vi "Run.vi"(8 "error in (no error)":errorcluster, 11 "Event in":refnum<class "Event.lvclass">) -> (0 "error out":errorcluster, 3 "Event out":refnum<class "Event.lvclass">)   [LabVIEW 2012, in "MDSplus.lvlib" / "Event.lvclass"]
doc: "Method run is called upon reception of the event with the associated name, specified in the constructor. The default implementation is void, and it will be likely overridden by subclasses."
uses:
  <vilib>/MDSplus/Classes/Event_Class/Event.lvclass
  <vilib>/MDSplus/MDSobjectsLVShr_64.dll
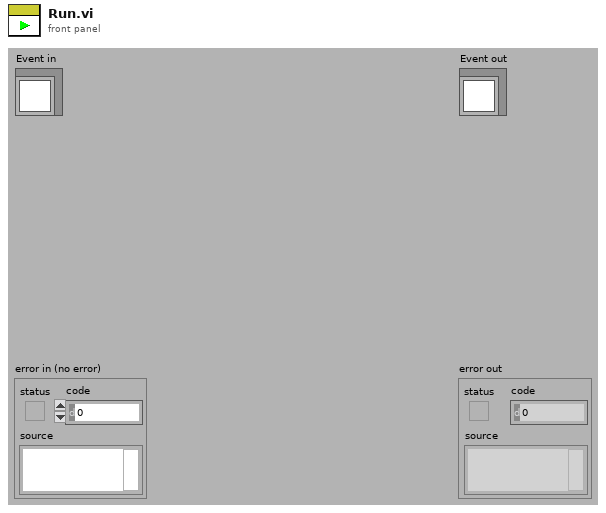
[diagram p1: front panel]
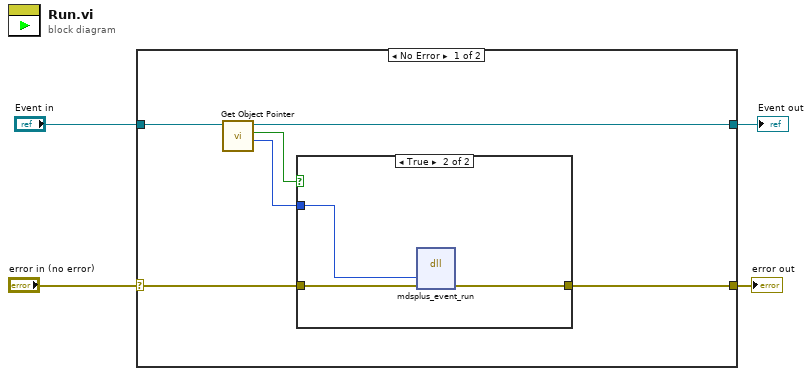
[diagram p0: block diagram]
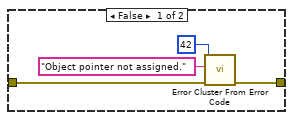
[diagram p2: hidden frame]
diagram:
  n1 = case shown="No Error" "error in (no error)" {
    selector: "error in (no error)" -> [w7 w19]
    tunnel: [w8 w19] -> w3
    tunnel: [w9 w18] -> w1
    tunnel: "Event in" -> [w10 w18]
    frame No Error {
      n2 = call-dynamic "Get Object Pointer.vi"("Event in"=w10) -> ("Object Pointer"=w5:i64, "Assigned object pointer?"=w6:bool, "Event out"=w9:refnum<class "Event.lvclass">)  [unwired: 8 in]
      n3 = case shown="True" w6 {
        tunnel: [w11 w17] -> w8
        tunnel: w7 -> [w12 w16]
        tunnel: w5 -> [_ w15]
        frame False {
          n4 = call <vilib>:"Error Cluster From Error Code.vi"("error in (no error)"=w12, "error message (\"\")"="Object pointer not assigned." ("error message (\"\")"), "error code (0)"=42) -> ("error out"=w11:errorcluster)  [unwired: 6 in]
        }
        frame True {
          n5 = dll-call lib="C:/Program Files/National Instruments/LabVIEW 2010/vi.lib/MDSplus/MDSobjectsLVShr**.*" fn="mdsplus_event_run"("lvEventPtr"=w15, "error"=w16) -> ("error"=w17:errorcluster)  [unwired: 5 in, 2 out]
        }
      }
    }
    frame Error {
    }
  }
  "error out" <- w3
  "Event out" <- w1
